vi "esp301 set enable.vi"(7 "Seperator in":string, 8 "error in (no error)":errorcluster, 9 "Args":string[](array[string]), 10 "String":string, 11 "ESP301 in":refnum<class "ESP301.lvclass">) -> (0 "error out":errorcluster, 2 "new commands":string, 3 "ESP301 out":refnum<class "ESP301.lvclass">)   [LabVIEW 2020, in "ESP301.lvclass"]
uses:
  ESP301.lvclass
  shared/OnOffTypeDef.ctl
  ESP301.lvclass/ESP301.ctl
  shared/CompressAndUpdate(Poly)/CompressAndUpdate(Enum).vi
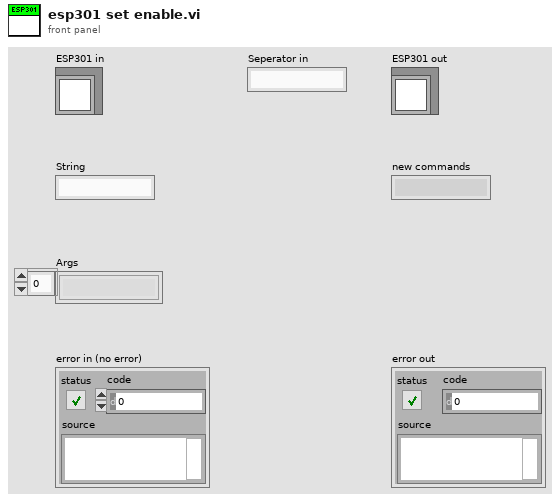
[diagram p1: front panel]
types:
  T1 = typedef "OnOffTypeDef.ctl" = enum16{"off", "on"}
  T2 = typedef "ESP301.lvclass/SettingsTypdef.ctl" = cluster{"devport":string, "Position":cluster{"Axis 1":cluster{"Value":dbl, "Min":dbl, "Max":dbl, "StepSize":dbl, "Tolerance":dbl, "ValueActual":dbl}, "Axis 2":cluster{"Value":dbl, "Min":dbl, "Max":dbl, "StepSize":dbl, "Tolerance":dbl, "ValueActual":dbl}, "Axis 3":cluster{"Value":dbl, "Min":dbl, "Max":dbl, "StepSize":dbl, "Tolerance":dbl, "ValueActual":dbl}}, "Power":cluster{"Axis 1":T1, "Axis 2":T1, "Axis 3":T1}, "Status":cluster{"Axis 1":T3, "Axis 2":T3, "Axis 3":T3}, "Backlash":cluster{"Axis 1":cluster{"Value":dbl, "Min":dbl, "Max":dbl, "StepSize":dbl, "Tolerance":dbl, "ValueActual":dbl}, "Axis 2":cluster{"Value":dbl, "Min":dbl, "Max":dbl, "StepSize":dbl, "Tolerance":dbl, "ValueActual":dbl}, "Axis 3":cluster{"Value":dbl, "Min":dbl, "Max":dbl, "StepSize":dbl, "Tolerance":dbl, "ValueActual":dbl}}, "Home":cluster{"Axis 1":cluster{"Value":dbl, "Min":dbl, "Max":dbl, "StepSize":dbl, "Tolerance":dbl, "ValueActual":dbl}, "Axis 2":cluster{"Value":dbl, "Min":dbl, "Max":dbl, "StepSize":dbl, "Tolerance":dbl, "ValueActual":dbl}, "Axis 3":cluster{"Value":dbl, "Min":dbl, "Max":dbl, "StepSize":dbl, "Tolerance":dbl, "ValueActual":dbl}}, "MoveToHardLimit":cluster{"Axis 1":T4, "Axis 2":T4, "Axis 3":T4}, "relativeMove":cluster{"Axis 1neg":T1, "Axis 2neg":T1, "Axis 3neg":T1, "Axis 1pos":T1, "Axis 2pos":T1, "Axis 3pos":T1}, "stepsize":cluster{"Value":dbl, "Min":dbl, "Max":dbl, "StepSize":dbl, "Tolerance":dbl, "ValueActual":dbl}, "automotoroff":T1, "ResetBeforeMove":T1, "Enable":cluster{"Axis 1":T1, "Axis 2":T1, "Axis 3":T1}, "InitWithDBValues":T1}
  T3 = typedef "status_TypDef.ctl" = enum16{"Not referenced", "Homing", "Moving", "Ready"}
  T4 = typedef "Hardware limit.ctl" = enum16{"pos", "neg"}
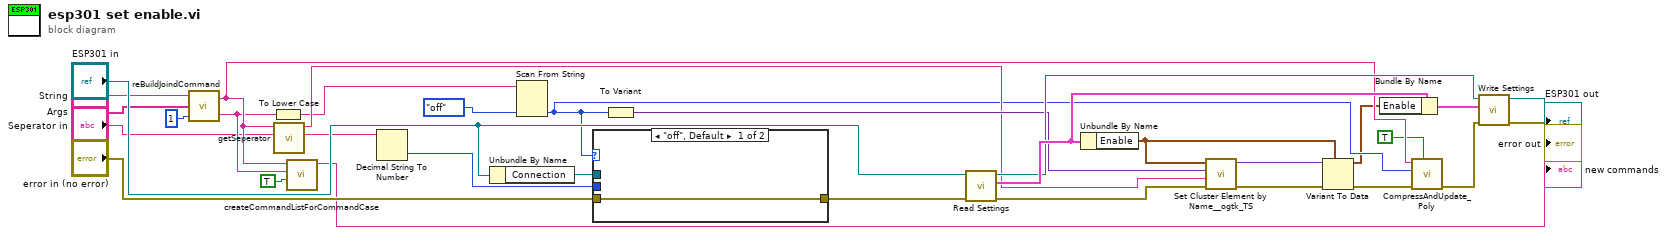
[diagram p0: block diagram]
diagram:
  n1 = call "reBuildJoindCommand.vi"("number of group elements (0)"=1, "Args"="Args", "Command 2"="String") -> ("Arg"=w15:string, "Command"=w22:string)
  n2 = To Lower Case(string=w15) -> (all lower case string=w14:string)
  n3 = call "getSeperator.vi"("Channel Seperator (\"\")"="Seperator in", "Command"=w22) -> ("Channel"=w8:string, "Seperator (e.g. \"Channel1\")"=w21:string)  [unwired: 8 in]
  n4 = call "createCommandListForCommandCase.vi"("immediate Check (only once)"=TRUE, "setvalue"=w15, "command"=w22) -> ("new commands"=→"new commands":string)  [unwired: 8 in]
  n5 = Decimal String To Number(string=w8) -> (number=w18:i32)  [unwired: 2 in, 1 out]
  n6 = Unbundle By Name("ESP301 in") -> ("Connection"=w19:refnum<visa-resource-name>)
  n7 = Scan From String(input string=w14, default 1=OnOffTypeDef."off" ("Axis 1")) -> (output 1=w17:T1)  [unwired: 3 in, 3 out]
  n8 = case shown="\"off\", Default" w17 {
    tunnel: w18 -> [_ _]
    tunnel: w19 -> [_ _]
    tunnel: [w33 w34] -> w30
    tunnel: "error in (no error)" -> [w33 w34]
    frame "off", Default {
    }
    frame "on" {
    }
  }
  n9 = To Variant(anything=w17) -> (Variant=w23:variant)
  n10 = call-dynamic "Read Settings.vi"("error in (no error)"=w30, "ESP301 in"="ESP301 in") -> ("error out"=w29:errorcluster, "Settings"=w28:T2, "ESP301 out"=w25:refnum<class "ESP301.lvclass">)  [unwired: 7 in]
  n11 = Unbundle By Name(w28) -> ("Enable"=w11:cluster{"Axis 1":T1, "Axis 2":T1, "Axis 3":T1})
  n12 = call "Set Cluster Element by Name__ogtk_TS.vi"("error in (no error)"=w29, "Element Name (\"\": New Element Data Name)"=w21, "New Element Value"=w23, "Cluster"=w11) -> ("error out"=w9:errorcluster, "VCluster out"=w10:variant)  [unwired: 5 in, 1 out]
  n13 = Variant To Data(error in=w9, type=w11, Variant=w10) -> (data=w12:cluster{"Axis 1":T1, "Axis 2":T1, "Axis 3":T1}, error out=w13:errorcluster)
  n14 = Bundle By Name(cluster=w28, "Enable"=w12) -> (w27:T2)
  n15 = call-poly "CompressAndUpdate_Poly.vi"("force CVT update (false)"=TRUE ("force CVT update"), "error in"=w13, "enum variant"=w17, "command or variable name"=w22) -> ("error out"=w31:errorcluster)  [unwired: 7 in]
  n16 = call-dynamic "Write Settings.vi"("error in (no error)"=w31, "Settings"=w27, "ESP301 in"=w25) -> ("error out"=→"error out":errorcluster, "ESP301 out"=→"ESP301 out":refnum<class "ESP301.lvclass">)  [unwired: 7 in]
